vi "WritebyWeakRefBoolArrS.vi"(8 "error in":errorcluster caption="entrée d'erreur", 10 "Valeur":bool, 11 "Control Ref":refnum<vi>[](array[refnum])) -> (0 "error out":errorcluster caption="sortie d'erreur")   [LabVIEW 2019]
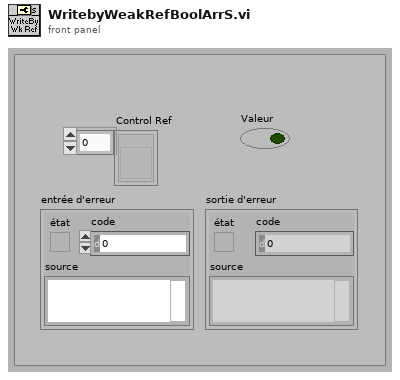
[diagram p1: front panel]
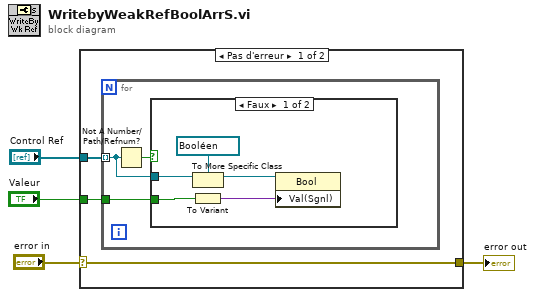
[diagram p0: block diagram]
diagram:
  n1 = case shown="Pas d'erreur" "error in" {
    selector: "error in" -> [w5 w16]
    tunnel: "Control Ref" -> [w7 _]
    tunnel: "Valeur" -> [w6 _]
    tunnel: [w5 w16] -> w1
    frame No Error {
      n2 = for {
        tunnel: w7 -> [w9] mode=indexing
        tunnel: w6 -> [w8]
        n3 = Not A Number/Path/Refnum?(number/path/refnum=w9) -> (NaN/Path/Refnum?=w10:bool)
        n4 = case shown="Faux" w10 {
          tunnel: w9 -> [w13 _]
          tunnel: w8 -> [w15 _]
          frame False {
            n5 = To More Specific Class(target class=refnum<vi> refnum ("référence"), reference=w13) -> (specific class reference=w12:refnum<vi>)  [unwired: 1 in, 1 out]
            n6 = To Variant(anything=w15) -> (Variant=w11:variant)
            n7 = property class="Bool"(reference=w12, "Val(Sgnl)"=w11) -> ()  [unwired: 1 in, 2 out]
          }
          frame True {
          }
        }
      }
    }
    frame Error {
    }
  }
  "error out" <- w1
